vi "Logging Read Var.vi"(4 "error in (no error)":errorcluster, 7 "LoggingDevRef":T1) -> (0 "error out":errorcluster, 1 "Output":T2, 2 "EOF":bool, 3 "LoggingDevRef":T1)   [LabVIEW 2012, in "femtoRoboLib.lvlib"]
uses:
  femtoRoboLib.lvlib
  Log Entry.ctl
  Log Value Type.ctl
  Log Value Cluster.ctl
  LoggingDevRef.ctl
  Log Entry - Converted.ctl
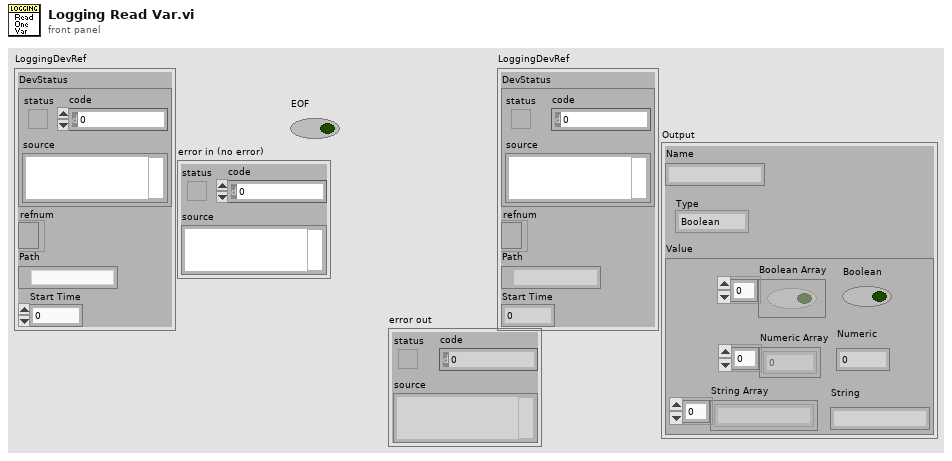
[diagram p1: front panel]
types:
  T1 = typedef "femtoRoboLib.lvlib/LoggingDevRef.ctl" = cluster{"DevStatus":errorcluster, "refnum":refnum<file>, "Path":path, "Start Time":u32}
  T2 = typedef "femtoRoboLib.lvlib/Log Entry.ctl" = cluster{"Name":string, "Type":T3, "Value":T4}
  T3 = typedef "femtoRoboLib.lvlib/Log Value Type.ctl" = enum16{"Boolean", "Numeric", "String", "Boolean Array", "Numeric Array", "String Array"}
  T4 = typedef "femtoRoboLib.lvlib/Log Value Cluster.ctl" = cluster{"Boolean Array":bool[], "Boolean":bool, "Numeric Array":dbl[], "Numeric":dbl, "String Array":string[], "String":string}
  T5 = typedef "femtoRoboLib.lvlib/Log Entry - Converted.ctl" = cluster{"Name":string, "Type":enum16{"Boolean", "Numeric", "String", "Boolean Array", "Numeric Array", "String Array"}, "Value":string}
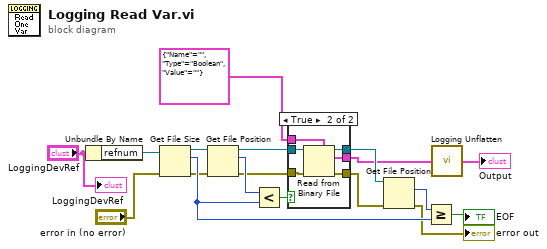
[diagram p0: block diagram]
diagram:
  n1 = Unbundle By Name("LoggingDevRef") -> ("refnum"=w9:refnum<file>)
  n2 = Get File Size(file=w9, error in="error in (no error)") -> (refnum out=w18:refnum<file>, size (in bytes)=w10:i64, 0:w6:errorcluster)
  n3 = Get File Position(4:w6, 7:w18) -> (0:w5:errorcluster, 2:w16:i64, 3:w13:refnum<file>)
  n4 = Less?(x=w16, y=w10) -> (x < y?=w15:bool)
  n5 = case shown="True" w15 {
    tunnel: T5 {"Name"="", "Type"=enum."Boolean", "Value"=""} ("Variable 2") -> [w21 w27]
    tunnel: [w21 w26] -> w2
    tunnel: [w20 w25] -> w14
    tunnel: w13 -> [w20 w22]
    tunnel: w5 -> [w19 w24]
    tunnel: [w19 w23] -> w4
    frame False {
    }
    frame True {
      n6 = Read from Binary File(5:w27, 8:w24, 11:w22) -> (0:w23:errorcluster, 2:w26:T5, 3:w25:refnum<file>)  [unwired: 3 in, 1 out]
    }
  }
  n7 = Get File Position(4:w4, 7:w14) -> (0:→"error out":errorcluster, 2:w11:i64)  [unwired: 1 out]
  n8 = Greater Or Equal?(x=w11, y=w10) -> (x >= y?=→"EOF":bool)
  n9 = call "Logging Unflatten.vi"("In"=w2) -> ("Out"=→"Output":T2)
  "LoggingDevRef" <- "LoggingDevRef"
